vi "CoordinatesCorrection.vi"(11 "Coordinates In":T1) -> (3 "Corrected Out":T1)   [LabVIEW 2020]
doc: "Converts the cursor position to the preview icon pixel position."
uses:
  <vilib>/Utility/miscctls.llb/LVPoint32TypeDef.ctl
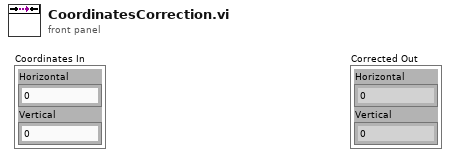
[diagram p1: front panel]
types:
  T1 = typedef "LVPoint32TypeDef.ctl" = cluster{"Horizontal":i32, "Vertical":i32}
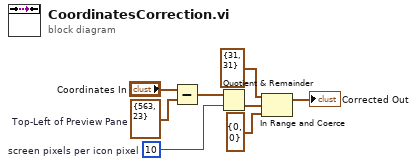
[diagram p0: block diagram]
diagram:
  w6 = 10  # screen pixels per icon pixel
  w8 = T1 {"Horizontal"=563, "Vertical"=23}  # Top-Left of Preview Pane
  n1 = Subtract(x="Coordinates In", y=w8) -> (x-y=w7:T1)
  n2 = Quotient & Remainder(x=w7, y=w6) -> (floor(x/y)=w5:T1)  [unwired: 1 out]
  n3 = In Range and Coerce(upper limit=T1 {"Horizontal"=31, "Vertical"=31}, x=w5, lower limit=T1 {"Horizontal"=0, "Vertical"=0}) -> (coerced(x)=→"Corrected Out":T1)  [unwired: 1 out]
